vi "PQcopySelect.vi"(6 "error in (no error)":errorcluster, 7 "CountClumn":string="id", 8 "optional clause":string, 9 "columns":string[](array[string]), 10 "table":string, 11 "conn":u32) -> (0 "database_status_message":T1, 1 "data":string[][](array[string]), 2 "column_names":string[](array[string]), 3 "conn_out":u32, 4 "error out":errorcluster)   [LabVIEW 2019, in "libpqutility64.lvlib"]
doc: "SELECT string gets embedded into COPY cmd and executed. Make shure to set CountColumn to initialise Resultset Array of LabVIEW. You might use an indexed Column for this."
uses:
  libpqutility64.lvlib
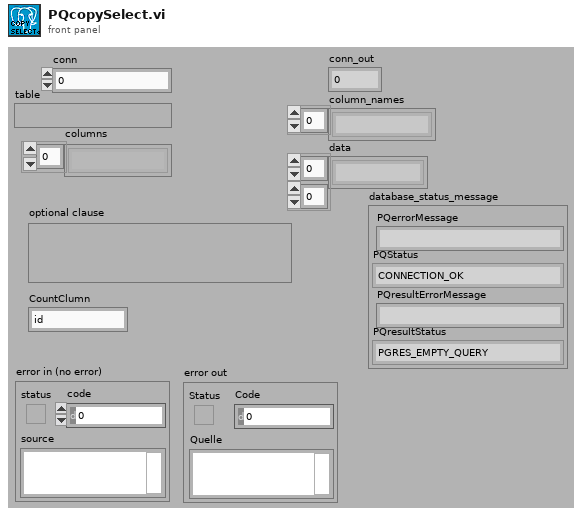
[diagram p1: front panel]
types:
  T1 = cluster{"PQerrorMessage":string, "PQStatus":enum16{"CONNECTION_OK", "CONNECTION_BAD", "CONNECTION_STARTED", "CONNECTION_MADE", "CONNECTION_AWAITING_RESPONSE", "CONNECTION_AUTH_OK", "CONNECTION_SETENV", "CONNECTION_SSL_STARTUP", "CONNECTION_NEEDED"}, "PQresultErrorMessage":string, "PQresultStatus":enum16{"PGRES_EMPTY_QUERY", "PGRES_COMMAND_OK", "PGRES_TUPLES_OK", "PGRES_COPY_OUT", "PGRES_COPY_IN", "PGRES_BAD_RESPONSE", "PGRES_NONFATAL_ERROR", "PGRES_FATAL_ERROR"}}
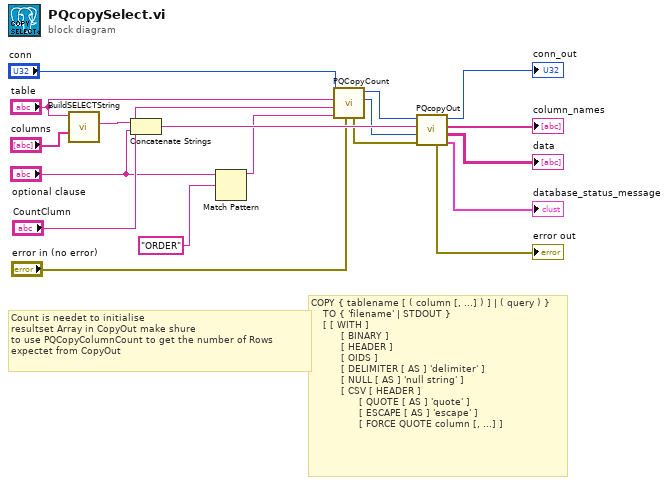
[diagram p0: block diagram]
diagram:
  # "Count is needet to initialise\nresultset Array in CopyOut make shure\nto use PQCopyColumnCount to get the number of Rows\nexpectet from CopyOut"
  # "COPY { tablename [ ( column [, ...] ) ] | ( query ) }\n    TO { 'filename' | STDOUT }\n    [ [ WITH ] \n          [ BINARY ]\n          [ HEADER ]\n          [ OIDS ]\n          [ DELIMITER [ AS ] 'delimiter' ]\n          [ NULL [ AS ] 'null string' ]\n          [ CSV [ HEADER ]\n                [ QUOTE [ AS ] 'quote' ] \n                [ ESCAPE [ AS ] 'escape' ]\n                [ FORCE QUOTE column [, ...] ]"
  n1 = call "BuildSELECTString.vi"("columns"="columns", "table"="table") -> ("select query"=w17:string)  [unwired: 9 in]
  n2 = Concatenate Strings(w17, "optional clause") -> (w11:string)
  n3 = Match Pattern(string="optional clause", regular expression="ORDER" ("Regulärer Ausdruck")) -> (before substring=w1:string)  [unwired: 1 in, 3 out]
  n4 = call "PQCopyCount.vi"("error in (no error)"="error in (no error)", "optional clause"=w1, "CountClumn"="CountClumn", "table"="table", "conn"="conn") -> ("Count"=w6:i32, "conn_out"=w9:u64, "error out"=w4:errorcluster)  [unwired: 3 in, 1 out]
  n5 = call "PQcopyOut.vi"("error in (no error)"=w4, "count"=w6, "query"=w11, "conn"=w9) -> ("database_status_message"=→"database_status_message":T1, "data"=→"data":string[][], "column_names"=→"column_names":string[], "conn_out"=→"conn_out":u32, "error out"=→"error out":errorcluster)  [unwired: 3 in]
